vi "读取VISA.vi"(8 "error in (no error)":errorcluster caption="错误输入（无错误）", 11 "多功能校准源接口输入":refnum<class "多功能校准源接口.lvclass">) -> (0 "error out":errorcluster caption="错误输出", 2 "VISA":refnum<visa-resource-name>, 3 "多功能校准源接口输出":refnum<class "多功能校准源接口.lvclass">)   [LabVIEW 2020, in "多功能校准源接口.lvlib" / "多功能校准源接口.lvclass"]
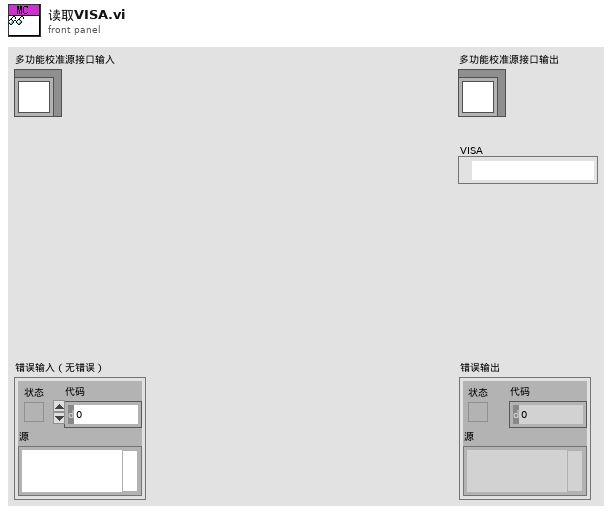
[diagram p1: front panel]
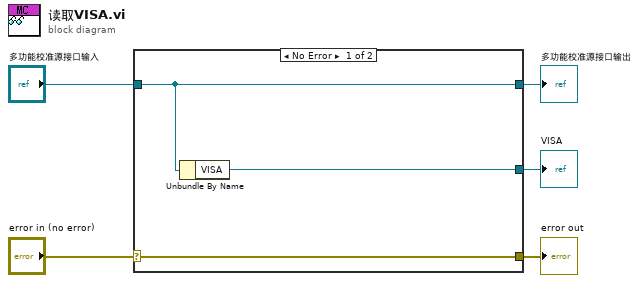
[diagram p0: block diagram]
diagram:
  n1 = case shown="No Error" "error in (no error)" {
    selector: "error in (no error)" -> [w8 w9]
    tunnel: [w8 w9] -> w4
    tunnel: [w7 w10] -> w2
    tunnel: "多功能校准源接口输入" -> [w7 w10]
    tunnel: [w6 _] -> w1
    frame No Error {
      n2 = Unbundle By Name(w7) -> ("VISA"=w6:refnum<visa-resource-name>)
    }
    frame Error {
    }
  }
  "error out" <- w4
  "多功能校准源接口输出" <- w2
  "VISA" <- w1
